vi "CTRE_Phoenix_MotorControl_Set.vi"(8 "error in (no error)":errorcluster, 9 "Output":dbl, 10 "Control Mode":T1 items=["PercentOutput"=0, "Position"=1, "Velocity"=2, "Current"=3, "Follower"=5, "MotionProfile"=6, "MotionMagic"=7, "MotionMagicArc"=8, "MotionProfileArc"=10, "Disabled"=15], 11 "PhoenixMotorControlDevRef":T2={"DeviceStatus"={"status"=FALSE, "code"=0, "source"=""}, "Type"=enum."PWM", "PWM"={"PWM Channel"=enum."PWM 1", "DeadBand"={"Name"="", "maxPositivePwm"=0, "minPositivePwm"=0, "centerPwm"=0, "maxNegativePwm"=0, "minNegativePwm"=0, "angularRange"=0}}, "CAN"={"Device Number"=0, "SetOutput VI Ref"=variant(enum8{"Percent VBus", "Current", "Speed", "Position", "Voltage"} enum."Percent VBus"), "GetOutput VI Ref"=variant(refnum<k1> refnum), "Enable VI Ref"=variant(dbl 12.0), "Disable VI Ref"=variant(enum8{"Percent VBus", "Speed", "Position", "Slave", "Unchanged / Invalid", "Voltage Compensation", "Current", "Motion Profile"} enum."Percent VBus"), "Data"=variant}, "Invert"=FALSE, "DIO PWM"={"PWM \"Enable\" Channel"=enum."Invalid", "DIOChannel"=enum."Invalid", "PWM Rate"=0.0}}) -> (0 "error out":errorcluster, 3 "PhoenixMotorControlDevRef":T2={"DeviceStatus"={"status"=FALSE, "code"=0, "source"=""}, "Type"=enum."PWM", "PWM"={"PWM Channel"=enum."PWM 1", "DeadBand"={"Name"="", "maxPositivePwm"=0, "minPositivePwm"=0, "centerPwm"=0, "maxNegativePwm"=0, "minNegativePwm"=0, "angularRange"=0}}, "CAN"={"Device Number"=0, "SetOutput VI Ref"=variant(enum8{"Percent VBus", "Current", "Speed", "Position", "Voltage"} enum."Percent VBus"), "GetOutput VI Ref"=variant(refnum<k1> refnum), "Enable VI Ref"=variant(dbl 12.0), "Disable VI Ref"=variant(enum8{"Percent VBus", "Speed", "Position", "Slave", "Unchanged / Invalid", "Voltage Compensation", "Current", "Motion Profile"} enum."Percent VBus"), "Data"=variant}, "Invert"=FALSE, "DIO PWM"={"PWM \"Enable\" Channel"=enum."Invalid", "DIOChannel"=enum."Invalid", "PWM Rate"=0.0}})   [LabVIEW 2017]
doc: "Sets the Output and Control Mode of the Motor Controller.\n\nIf setting the controller to \"Follower\" mode, the output value should be the Master Device Number."
uses:
  <vilib>/Rock Robotics/WPI/MotorControl/WPI_MotorControlDeviceRef.ctl
  <vilib>/Rock Robotics/WPI/MotorControl/WPI_MotorControlType.ctl
  <vilib>/Rock Robotics/SystemInterfaces/DIO/FPGA_DIOPWMChannel.ctl
  <vilib>/Rock Robotics/WPI/PWM/WPI_PWMDeadband.ctl
  <vilib>/Rock Robotics/SystemInterfaces/DIO/FPGA_DIOChannel.ctl
  Controls/CTRE_Phoenix_MotorControl_ControlMode.ctl
  Controls/CTRE_Phoenix_MotorControl_DevRefData.ctl
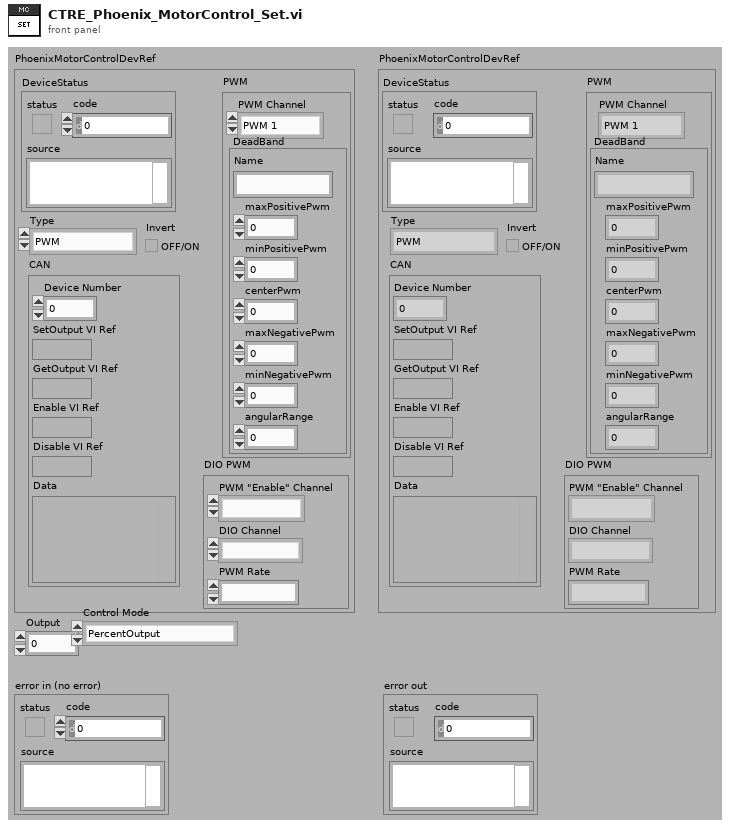
[diagram p1: front panel]
types:
  T1 = typedef "CTRE_Phoenix_MotorControl_ControlMode.ctl" = u16
  T2 = typedef "WPI_MotorControlDeviceRef.ctl" = cluster{"DeviceStatus":errorcluster, "Type":T3, "PWM":cluster{"PWM Channel":T4, "DeadBand":T5}, "CAN":cluster{"Device Number":u8, "SetOutput VI Ref":variant, "GetOutput VI Ref":variant, "Enable VI Ref":variant, "Disable VI Ref":variant, "Data":variant}, "Invert":bool, "DIO PWM":cluster{"PWM \"Enable\" Channel":T4, "DIOChannel":T6, "PWM Rate":dbl}}
  T3 = typedef "WPI_MotorControlType.ctl" = enum16{"PWM", "CAN", "DIO PWM"}
  T4 = typedef "FPGA_DIOPWMChannel.ctl" = enum8{"PWM 0", "PWM 1", "PWM 2", "PWM 3", "PWM 4", "PWM 5", "PWM 6", "PWM 7", "PWM 8", "PWM 9", "PWM MXP 0", "PWM MXP 1", "PWM MXP 2", "PWM MXP 3", "PWM MXP 4", "PWM MXP 5", "PWM MXP 6", "PWM MXP 7", "PWM MXP 8", "PWM MXP 9", "Invalid"}
  T5 = typedef "WPI_PWMDeadband.ctl" = cluster{"Name":string, "maxPositivePwm":i32, "minPositivePwm":i32, "centerPwm":i32, "maxNegativePwm":i32, "minNegativePwm":i32, "angularRange":u16}
  T6 = typedef "FPGA_DIOChannel.ctl" = enum8{"DIO 0", "DIO 1", "DIO 2", "DIO 3", "DIO 4", "DIO 5", "DIO 6", "DIO 7", "DIO 8", "DIO 9", "DIO MXP 0", "DIO MXP 1", "DIO MXP 2", "DIO MXP 3", "DIO MXP 4", "DIO MXP 5", "DIO MXP 6", "DIO MXP 7", "DIO MXP 8", "DIO MXP 9", "DIO MXP 10", "DIO MXP 11", "DIO MXP 12", "DIO MXP 13", "DIO MXP 14", "DIO MXP 15", "SPI Port CS1", "SPI Port CS2", "SPI Port CS3", "SPI Port MISO", "SPI Port MOSI", "Invalid"}
  T7 = typedef "CTRE_Phoenix_MotorControl_DevRefData.ctl" = cluster{"Library":path, "handle":u64, "Control Mode":T1, "UsageFrame":u32, "RefNumName":string, "arbID":u32}
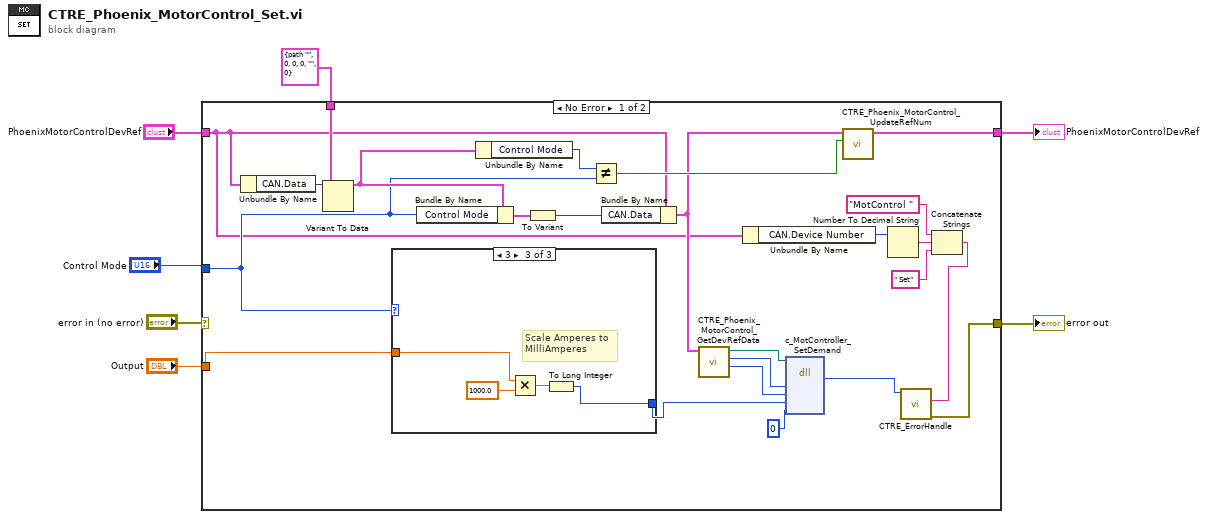
[diagram p0: block diagram]
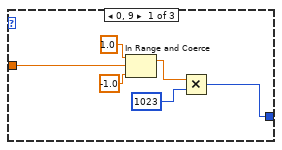
[diagram p2: hidden frame]
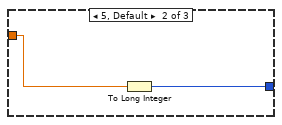
[diagram p3: hidden frame]
diagram:
  n1 = case shown="No Error" "error in (no error)" {
    selector: "error in (no error)" -> [_ w45]
    tunnel: [w8 w45] -> w7
    tunnel: [w26 w44] -> w5
    tunnel: "PhoenixMotorControlDevRef" -> [w11 w44]
    tunnel: "Control Mode" -> [w23 _]
    tunnel: "Output" -> [w31 _]
    tunnel: T7 {"Library"=path "", "handle"=0, "Control Mode"=0, "UsageFrame"=0, "RefNumName"="", "arbID"=0} ("Cluster") -> [w30 _]
    frame No Error {
      n2 = Unbundle By Name(w11) -> ("CAN.Data"=w27:variant)
      n3 = Variant To Data(type=w30, Variant=w27) -> (data=w25:T7)  [unwired: 1 in, 1 out]
      n4 = case shown="3" w23 {
        tunnel: [w33 w38 w42] -> w16
        tunnel: w31 -> [w32 w39 w41]
        frame 0, 9 {
          n5 = In Range and Coerce(upper limit=1.0, x=w32, lower limit=-1.0) -> (coerced(x)=w35:dbl)  [unwired: 1 out]
          n6 = Multiply(x=w35, y=u32 1023) -> (x*y=w33:i32)
        }
        frame 5, Default {
          n7 = To Long Integer(number=w39) -> (32bit integer=w38:i32)
        }
        frame 3 {
          # "Scale Amperes to\nMilliAmperes"
          n8 = Multiply(x=w41, y=1000.0) -> (x*y=w43:dbl)
          n9 = To Long Integer(number=w43) -> (32bit integer=w42:i32)
        }
      }
      n10 = Bundle By Name(cluster=w25, "Control Mode"=w23) -> (w28:T7)
      n11 = Unbundle By Name(w25) -> ("Control Mode"=w24:T1)
      n12 = To Variant(anything=w28) -> (Variant=w29:variant)
      n13 = Not Equal?(x=w24, y=w23) -> (x != y?=w22:bool)
      n14 = Bundle By Name(cluster=w11, "CAN.Data"=w29) -> (w21:T2)
      n15 = call "CTRE_Phoenix_MotorControl_GetDevRefData.vi"("PhoenixMotorControlDevRef"=w21) -> ("Talon SRX Mode"=w18:T1, "handle"=w19:u64, "Library"=w20:path)  [unwired: 4 in, 4 out]
      n16 = Unbundle By Name(w11) -> ("CAN.Device Number"=w15:u8)
      n17 = dll-call lib="?" fn="c_MotController_SetDemand"(path in=w20, "handle"=w19, "mode"=w18, "demand0"=w16, "demand1"=0) -> ("return type"=w9:i32)  [unwired: 6 in, 2 out]
      n18 = call "CTRE_Phoenix_MotorControl_UpdateRefNum.vi"("Update"=w22, "PhoenixMotorControlDevRef"=w21) -> ("PhoenixMotorControlDevRef"=w26:T2)  [unwired: 9 in]
      n19 = Number To Decimal String(number=w15) -> (decimal integer string=w14:string)  [unwired: 1 in]
      n20 = Concatenate Strings("MotControl " ("string"), w14, " Set" ("string")) -> (w10:string)
      n21 = call "CTRE_ErrorHandle.vi"("origin"=w10, "code"=w9) -> ("error out"=w8:errorcluster)  [unwired: 9 in]
    }
    frame Error {
    }
  }
  "PhoenixMotorControlDevRef" <- w5
  "error out" <- w7
